vi "String_Convert.vi"(1 "String Array":string[](array[string])) -> (0 "Numerical Array":dbl[](array[numeric]))   [LabVIEW 2019]
doc: "Convert an array of numerical strings to floats\n\nNaN values are excluded\n\nR. Sheehan 10 - 8 -2018"
panel:
  in  "index":i32
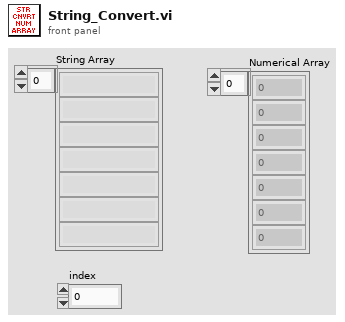
[diagram p1: front panel]
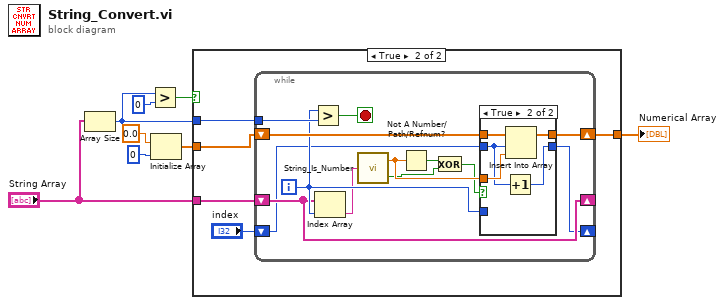
[diagram p0: block diagram]
diagram:
  n1 = Array Size(array="String Array") -> (size(s)=w2:i32)
  n2 = Greater?(x=w2, y=0) -> (0:w7:bool)
  n3 = Initialize Array(0.0 ("element"), 0 ("dimension size")) -> (w4:dbl[])
  n4 = case shown="True" w7 {
    tunnel: w4 -> [w9 w13]
    tunnel: [w9 w12] -> w3
    tunnel: w2 -> [_ w14]
    tunnel: "String Array" -> [_ w11]
    frame False {
    }
    frame True {
      n5 = while {
        tunnel: w14 -> [w27]
        shift-right: [w24] -> w12
        shift-left: w13 -> [w25]
        shift-right: [w21] -> _
        shift-left: w11 -> [w21]
        shift-right: [w19] -> _
        shift-left: "index" -> [w20]
        i -> [w23]
        stop <- w26 stop-if-true
        n6 = Greater?(x=w23, y=w27) -> (0:w26:bool)
        n7 = Index Array(array=w21, index=w23) -> (element=w22:string)
        n8 = call "String_Is_Number.vi"("String"=w22) -> ("Number"=w18:dbl, "Is Number?"=w16:bool)
        n9 = Not A Number/Path/Refnum?(number/path/refnum=w18) -> (NaN/Path/Refnum?=w17:bool)
        n10 = Exclusive Or(1:w16, 2:w17) -> (0:w15:bool)
        n11 = case shown="True" w15 {
          tunnel: w18 -> [_ w32]
          tunnel: w25 -> [w29 w34]
          tunnel: [w29 w33] -> w24
          tunnel: w23 -> [_ _]
          tunnel: w20 -> [w28 w31]
          tunnel: [w28 w30] -> w19
          frame False {
          }
          frame True {
            n12 = Increment(x=w31) -> (x+1=w30:i32)
            n13 = Insert Into Array(array=w34, index=w31, new element=w32) -> (w33:dbl[])
          }
        }
      }
    }
  }
  "Numerical Array" <- w3
